vi "GUI_Bella_Control_Center.vi"() -> ()   [LabVIEW 2020]
uses:
  Shared/GUI_Template/GUI_master/tcp_new_data_event.ctl
  Shared/GUI_Template/GUI_master/tcp new data cluster.ctl
  GUI_TestStand/Fire button.ctl
  Device Drivers/DG645/subVIs/TriggerSource_TypDef.ctl
  <vilib>/Utility/config.llb/Write Key (I32).vi
  <vilib>/Platform/browser.llb/Open URL in Default Browser (string).vi
  <vilib>/Analysis/NI_AALBase.lvlib
  <vilib>/Utility/config.llb/NI_LVConfig.lvlib
panel:
  in  "JetOnTime":dbl=0.001 format="%#_6p"
  in  "Position.Channel 3::25":dbl caption="SMFiber (35.6in, 1out)" min=1.0 max=50.0 format="%.1f"
  in  "GasJetOn":bool
  in  "SendExptCmds":bool
  in  "ShotControl":bool
  in  "Thales.DIAG_CU_Output_Percent_1::37":dbl caption="Amp2 att (%)" min=1.0 max=100.0 step=500.0 format="%.2f"
  in  "GUIdevice 37":string="SVE-LT-Thales"
  in  "Pressure.device 1::39":dbl caption="Backing pressure" min=0.0 max=314.0 format="%.3f"
  in  "GUIdevice 39":string="PRC-PL1-HighPressure"
  in  "Scan":T1(ring)
  in  "LogTable":bool
  in  "New Google\nExpLog for new day?":bool=TRUE
  out "standard output":string
  in  "Create Log":bool caption="LogTable"
  in  "GUIdevice 38":string="STAGE-2BL-Compressor"
  in  "Position.Axis 1::38":dbl caption="Comp2 Translation" min=0.0 max=20.0 format="%.3f"
  in  "Position.Channel 5::31":T2(ring) caption="FROG foil"
  in  "Position.Channel 2::31":T2(ring) caption="Little Rick"
  in  "AnalogOutput.Channel 1::36":dbl caption="M4A att (V)" min=0.0 max=5.0 step=500.0 format="%.2f"
  in  "GUIdevice 36":string="ATT-2BL-M4A"
  in  "GUIdevice 35":string="ATT-2BL-DM"
  in  "AnalogOutput.Channel 1::35":dbl caption="2BL DM att (V)" min=0.0 max=5.0 step=500.0 format="%.2f"
  in  "Step size 2":dbl=20.0 caption="Step size" min=-22.0 max=22.0
  in  "Position.Axis 4::34":dbl caption="OFI Holy V F8" min=-100000.0 max=100000.0 step=500.0
  in  "Position.Axis 3::34":dbl caption="OFI Holy H F7" min=-100000.0 max=100000.0 step=500.0
  in  "Position.Axis 2::34":dbl caption="Axicon V F6" min=-100000.0 max=100000.0 step=500.0
  in  "Position.Axis 1::34":dbl caption="Axicon H F5" min=-100000.0 max=100000.0 step=500.0
  in  "GUIdevice 34":string="MCD-PL1-picosOFI2"
  in  "Position.Axis 4::33":dbl caption="BesselM1 V F4" min=-100000.0 max=100000.0 step=500.0
  in  "Position.Axis 3::33":dbl caption="BesselM1 H F3" min=-100000.0 max=100000.0 step=500.0
  in  "Position.Axis 2::33":dbl caption="OFI Probe V F2" min=-100000.0 max=100000.0 step=500.0
  in  "Position.Axis 1::33":dbl caption="OFI Probe H F1" min=-100000.0 max=100000.0 step=500.0
  in  "GUIdevice 33":string="MCD-PL1-picosOFI1"
  in  "delay.Channel_B::32":dbl caption="jet open time" min=-0.1 max=0.1 format="%.3p"
  in  "delay.Channel_A::32":dbl caption="jet open" min=-0.1 max=0.1 format="%.3p"
  in  "GUIdevice 32":string="DDG-AA-SRSgasjet"
  in  "position::6":dbl caption="LPmode stage long (605 safe)" min=0.0 max=605.0 format="%.1f"
  in  "GUIdevice 6":string="STAGE-PL1-LPmodeLong"
  in  "EnableMotor::6":bool caption="LPmode motor \nstatus"
  in  "CapStatus":enum16{"out", "in", "Unknown"}(ring) caption="Cap"
  in  "position::4":dbl=-1.631e-06 caption="Capstage" min=0.0 max=600.0 format="%.1f"
  in  "GUIdevice 4":string="STAGE-PL1-Capstage1"
  out "Boolean 2":bool
  in  "GUIdevice 31":string="1WIRE-BELLA-Flipper"
  in  "Position.Channel 4::31":T2(ring) caption="PL1 Fiber"
  in  "Amplitude.Ch GH::10":dbl=-1.631e-06 caption="Shot Shutter V" min=0.5 max=5.0 format="%.1f"
  in  "Rate (Hz)":dbl=0.3
  out "Crystal2":enum16{"In", "Out", "Unknown"}(ring)
  out "Hex1posdesc":enum16{"guiding", "fiber ref", "Unknown"}(ring) caption="Hex1"
  in  "DigitalOutput.Channel 0::30":enum16{"off", "on"}(ring) caption="GVD Plunger"
  in  "GUIdevice 30":string="DAQ-PL1-GVD"
  in  "GUIdevice 29":string="MCD-HEAT-ESP0"
  in  "Position.Axis 2::29":dbl caption="Y" min=-5.0 max=25.0 format="%.4f"
  in  "Position.Axis 1::29":dbl caption="X" min=-5.0 max=25.0 format="%.4f"
  in  "wangle::28":dbl caption="w" min=-1.0 max=1.0 step=0.01 format="%.5f"
  in  "vangle::28":dbl caption="v" min=-5.0 max=5.0 step=0.01 format="%.5f"
  in  "uangle::28":dbl caption="u" min=-1.0 max=1.0 step=0.01 format="%.5f"
  in  "ypos::28":dbl caption="y" min=-2.0 max=8.0 step=0.01 format="%.5f"
  in  "zpos::28":dbl caption="z" min=-5.0 max=5.0 step=0.01 format="%.5f"
  in  "xpos::28":dbl caption="x" min=-0.5 max=0.5 step=0.01 format="%.5f"
  in  "GUIdevice 28":string="HEX-PL1-2"
  in  "delay.Channel_A::27":dbl caption="Disch timing both caps" min=-0.1 max=0.1 format="%.3p"
  out "Boolean":bool
  in  "amplitude.Channel_A::27":dbl caption="Caps Trig (V)" min=-3.0 max=4.0 format="%.2f"
  in  "GUIdevice 27":string="DDG-AA-SRS3"
  in  "GUIdevice 26":string="PRC-PL1-PressureAPL"
  in  "pressure::26":dbl caption="Cap2 Pressure (Torr)" min=0.0 max=50.0 format="%.2f"
  in  "Position.Channel 5::25":dbl caption="Wedge (43.5,2)" min=0.0 max=50.0 format="%.1f"
  in  "Position.Channel 4::25":dbl caption="ND2 (4,45)" min=-35.0 max=-12.0 format="%.1f"
  in  "Position.Channel 1::25":dbl caption="LPmode kicker (79in, 1out)" min=0.5 max=83.0 format="%.1f"
  in  "Position.Channel 2::25":dbl caption="XH (38.1,2)" min=0.0 max=30.0 format="%.1f"
  in  "Position.Channel 1::25":dbl caption="ND3 (4,45)" min=0.5 max=83.0 format="%.1f"
  out "Data.Channel 2::14":dbl caption="Flow US (sccm)" min=0.0 max=1000.0 format="%.1f"
  out "pressure2::5":dbl caption="PDR US (Torr)" min=-100.0 max=500.0 format="%.2f"
  in  "Data.Channel 2::11":dbl caption="Pressure US (Torr)" min=0.0 max=1000.0 format="%.2f"
  in  "GUIdevice 25":string="STAGE-PL1-Smaract"
  in  "Heater Alignment Directions":bool
  in  "Position.device 4::16":dbl caption="2Y" min=-40000000.0 max=40000000.0
  in  "Position.device 3::16":dbl caption="2X" min=-40000000.0 max=40000000.0
  in  "Position.device 2::16":dbl caption="1Y" min=-40000000.0 max=40000000.0
  in  "Position.device 1::16":dbl caption="1X" min=-40000000.0 max=40000000.0
  in  "Position.Axis 3::15":dbl caption="XY" min=-3.0 max=16.0 format="%.4f"
  in  "Position.Axis 2::15":dbl caption="Y" min=-3.0 max=17.0 format="%.4f"
  in  "Position.Axis 1::15":dbl caption="X" min=-3.0 max=13.0 format="%.4f"
  in  "GUIdevice 24":string="STAGE-HEAT-TL1"
  in  "Encoder position::23":dbl caption="position HPD2" min=0.0 max=600.0 format="%.1f"
  in  "position::3":dbl caption="position HPD" min=0.0 max=600.0 format="%.1f"
  in  "GUIdevice 23":string="STAGE-HPD-Far"
  in  "GUIdevice 22":string="MANPAR-BELLA-FireCont"
  in  "Allow Fire Continues":bool
  out "Fire continues Indicator":bool caption="firing"
  in  "Fire Button":T3=TRUE
  in  "Trigger.Source::10":T4 caption="SRS Trigger Mode"
  in  "value2::21":dbl=-1.631e-06 caption="Offset" min=-9999999.0 max=9999999.0 format="%.3p"
  in  "value1::21":dbl=-0.000129636 caption="Offset" min=-9999999.0 max=9999999.0 format="%#.4p"
  out "Absolute Heater timing":dbl caption="delay" format="%#.4p"
  out "Absolute discharge timing":dbl caption="delay from pk" format="%#.3p"
  in  "delay.Channel_A::19":dbl caption="Timing box" min=-0.1 max=0.1 format="%#.4p"
  in  "Delay.Ch E::17":dbl caption="Timing box" min=-0.1 max=0.1 format="%.3p"
  in  "value0::22":bool caption="Fire continuosly"
  in  "GUIdevice 21":string="MANPAR-BELLA-Timing"
  out "PWshutter Scanstart":string
  out "Heater Scanstart":string
  in  "position::18":enum16{"out", "in", "Unknown"}(ring) caption="Cap stage"
  in  "bigshuttermode::18":enum16{"Auto", "Manual"}(ring) caption="Heater shutter mode"
  in  "smallshuttermode::18":enum16{"Auto", "Manual"}(ring) caption="PW tel4 shutter mode"
  in  "smallshutterposition::18":enum16{"out", "in", "Unknown"}(ring) caption="PW tel4 shutter"
  in  "bigshutterposition::18":enum16{"out", "in", "Unknown"}(ring) caption="Heater shutter"
  in  "voltage::20":dbl caption="Discharge HV (kV)" min=0.0 max=40.0 format="%.2f"
  in  "GUIdevice 20":string="HV-PL1-Glassman"
  in  "SlaveValue::11":dbl caption="Slave Value (%)" min=0.0 max=200.0 format="%.1f"
  in  "Update offsets":bool caption="Update"
  in  "Offset Heater timing":dbl=-0.000129636 caption="Offset" format="%#.3p"
  in  "Offset discharge timing":dbl=-1.631e-06 caption="Offset" format="%#.3p"
  in  "GUIdevice 19":string="DDG-HEAT-SRS1"
  in  "GUIdevice 18":string="STAGE-PL1-Cap1"
  in  "GUIdevice 16":string="PICO-HEAT-1"
  in  "GUIdevice 15":string="MCD-HEAT-ESP1"
  in  "GUIdevice 17":string="DDG-AA-SRS0"
  out "error IO 2":errorcluster
  out "fire::10":string
  out "tcp data event":T5
  in  "UDP error message":string
  in  "GUIdevice 14":string="GAUGE-PL1-FlowStage1"
  in  "GUIdevice 13":string="DDG-AA-SRS2"
  in  "GUIdevice 7":string="MANPAR-PL1-BottlePressure"
  in  "parameter::2":string="parameter" caption="Manual parameter"
  in  "GUIdevice 2":string="MANPAR-BELLA-General"
  in  "GUIdevice 10":string="DDG-AA-ShotCntrl"
  in  "GUIdevice 5":string="GAUGE-PL1-Pressure"
  in  "GUIdevice 1":string="HEX-PL1-1"
  in  "GUIdevice 3":string="STAGE-HPD-Tel"
  in  "GUIdevice 11":string="PRC-PL1-Stage1"
  in  "Delay.Ch E::13":dbl caption="Discharge timing (s)" min=-0.1 max=0.2 format="%#_9p"
  out "Trans sigma":dbl format="%0.2f"
  out "Trans Mean":dbl format="%0.2f"
  out "Waveform Chart":dbl(graph)
  out "EnergyIn::2":dbl caption="Ein" min=0.0 max=0.0 format="%.1p"
  out "EnergyOut::12":dbl caption="Eout" min=0.0 max=0.0 format="%.1p"
  in  "EnergyTransmission::12":dbl caption="Etrans (%)" min=0.0 max=0.0
  in  "GUIdevice 12":string="EM-AA-Trans1"
  in  "<command>::1":bool caption="ABORT\nHEXAPOD"
  in  "Step size":dbl min=-22.0 max=22.0 format="%.5f"
  in  "wangle::1":dbl caption="w (F11 F12)" min=-6.0 max=6.0 step=0.01 format="%.5f"
  in  "vangle::1":dbl caption="v (F9 F10)" min=-6.0 max=6.0 step=0.01 format="%.5f"
  in  "uangle::1":dbl caption="u (F7 F8)" min=-6.0 max=6.0 step=0.01 format="%.5f"
  in  "ypos::1":dbl caption="y (F3 F4)" min=-20.0 max=10.0 step=0.01 format="%.5f"
  in  "zpos::1":dbl caption="z (PgU PgD)" min=-12.0 max=1.0 step=0.01 format="%.5f"
  in  "xpos::1":dbl caption="x (F1 F2)" min=-22.0 max=22.0 step=0.01 format="%.5f"
  in  "value::7":dbl caption="Bottle Pressure" min=0.0 max=1000.0
  in  "Pressure.device 1::6":dbl caption="Alicat Pressure" min=0.0 max=314.0 format="%.2f"
  in  "Position.Axis 1::9":dbl caption="Comp1 Translation" min=-50.0 max=50.0 format="%.3f"
  in  "GUIdevice 9":string="STAGE-1BL-Compression"
  out "Data.Channel 1::14":dbl caption="Flow DS (sccm)" min=0.0 max=1000.0 format="%.1f"
  in  "Data.Channel 1::11":dbl caption="Pressure DS (Torr)" min=0.0 max=1000.0 format="%.2f"
  out "pressure::5":dbl caption="PDR DS (Torr)" min=-100.0 max=500.0 format="%.2f"
  in  "Delay.Ch C::10":dbl caption="Jet timing (s)" min=-0.1 max=2.1 format="%#_6p"
  in  "stop":bool
  # "BELLA CONTROL CENTER"
  # "CAP"
  # "Hex2"
  # "HEXAPOD"
  # "PICOS"
  # "DG"
  # "HEXAPOD 2"
  # "Energy"
  # "GAS JET"
  # "Scan"
  # "Discharge timing (s)"
  # "Send only. Does not read"
  # "1wire"
  # "Jet"
  # "Heater timing (s)"
  # "\"-x\" is laser propagation direction"
  # "HPD Stage"
  # "PL1 stages"
  # "Heater Alignment"
  # "Atttenuate"
  # "Heat ESP0"
  # "Heat ESP1"
  # "Compressors"
  # "Heat Pico"
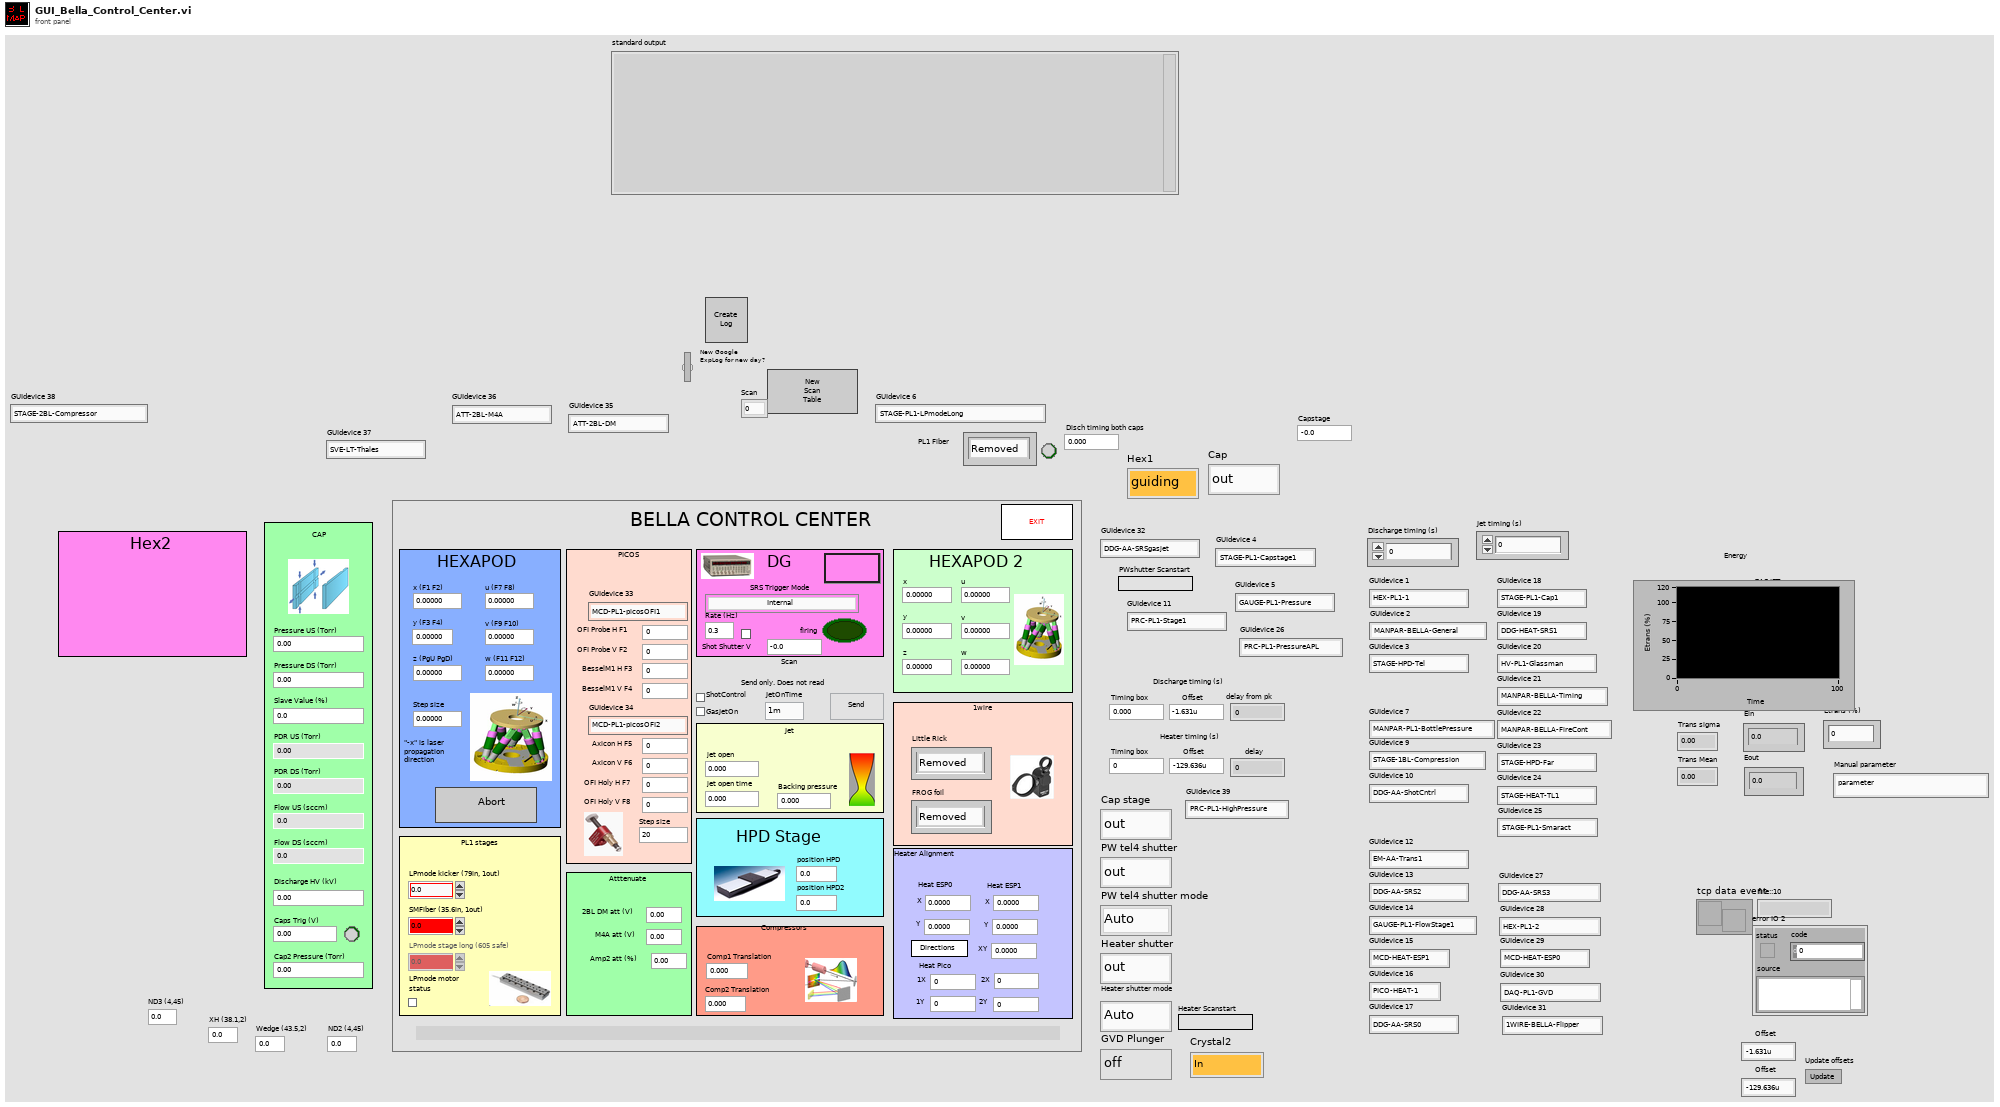
[diagram p1: front panel]
types:
  T1 = enum16{"0", "1", "2", "3", "4", "5", "6", "7", "8", "9", "10", "11", "12", "13", "14", "15", "16", "17", "18", "19", "20", "21", "22", "23", "24", "25", "26", "27", "28", "29", "30", "31", "32", "33", "34", "35", "36", "37", "38", "39", "40", "41", "42", "43", "44", "45", "46", "47", "48", "49", "50", "51", "52", "53", "54", "55", "56", "57", "58", "59", "60", "61", "62", "63", "64", "65", "66", "67", "68", "69", "70", "71", "72", "73", "74", "75", "76", "77", "78", "79", "81", "82", "83", "84", "85", "86", "87", "88", "89", "90", "91", "92", "93", "94", "95", "96", "97", "98", "99", ""}
  T2 = enum16{"Removed", "Inserted", "Unknown", "Moving"}
  T3 = typedef "Fire button.ctl" = bool
  T4 = typedef "TriggerSource_TypDef.ctl" = enum16{"Internal", "External rising edges", "External falling edges", "Single shot external rising edges", "Single shot external falling edges", "Single shot", "Line"}
  T5 = typedef "tcp_new_data_event.ctl" = refnum<user-event>
  T6 = typedef "tcp new data cluster.ctl" = cluster{"EventEnum":enum16{"new data", "connection status update"}, "Device name":string}
  T7 = enum8{"Enabled", "Disabled", "Disabled and Grayed Out"}
  T8 = enum32{"invalid app kind", "Development System", "Run Time System", "Student Edition", "Embedded LabVIEW", "Evaluation", "Custom"}
  T9 = enum32{"Invalid", "Standard", "Closed", "Hidden", "Minimized", "Maximized"}
  T10 = typedef "imagedata.ctl" = cluster{"image type":i32, "image depth":i32, "image":u8[], "mask":u8[], "colors":u32[], "Rectangle":cluster{"left":i16, "top":i16, "right":i16, "bottom":i16}}
  T11 = typedef "NI_LVConfig.lvlib/Config Data RefNum.ctl" = refnum<k1>
  T12 = cluster{"Core":cluster{"Current VI Reference":refnum<vi>, "Close Panel on Exit?":bool}, "Heater timing offset":dbl, "Discharge timing offset":dbl, "Jet trigger":bool, "Tik1":u32, "Tik2":u32, "Fire Continues Allowed":bool}
  T13 = cluster{"Current VI Reference":refnum<vi>, "Close Panel on Exit?":bool}
  T14 = typedef "mysql_authentication.ctl" = cluster{"User":string, "Password":string, "Database":string}
  T15 = cluster{"Port":u16, "IP Address":string, "Authentication":T14}
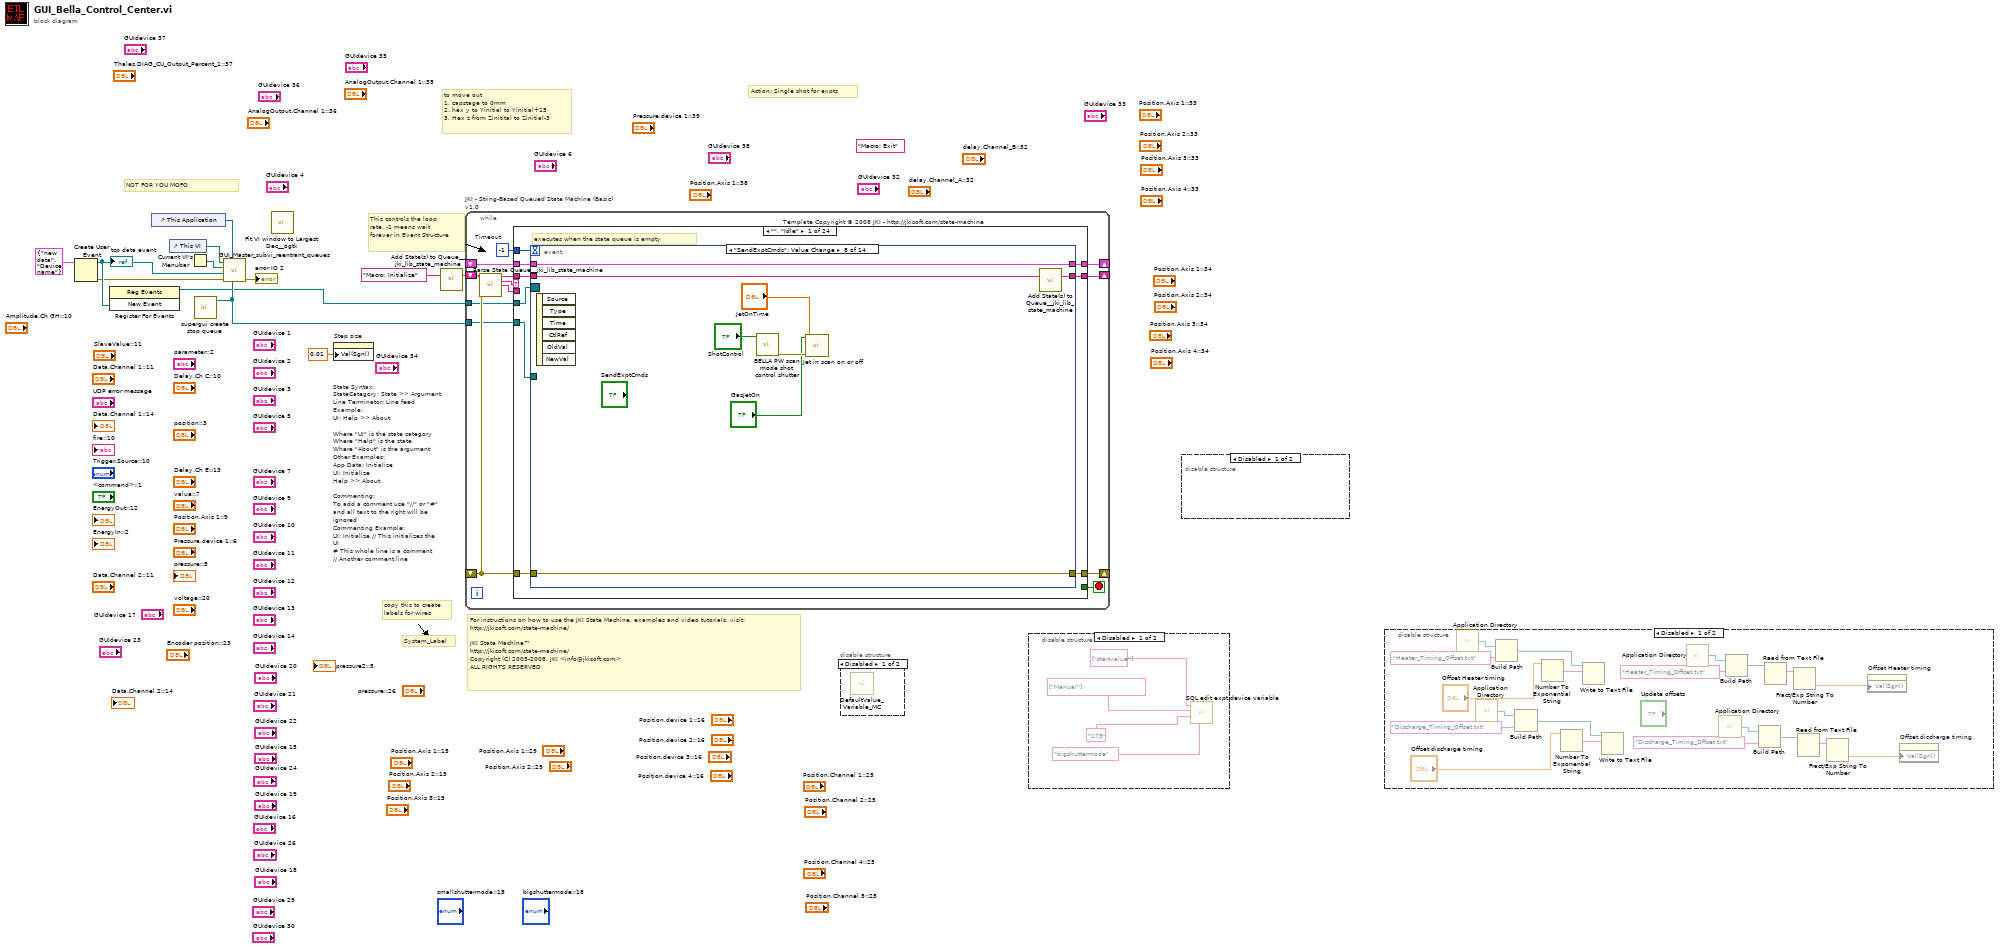
[diagram p0: block diagram]
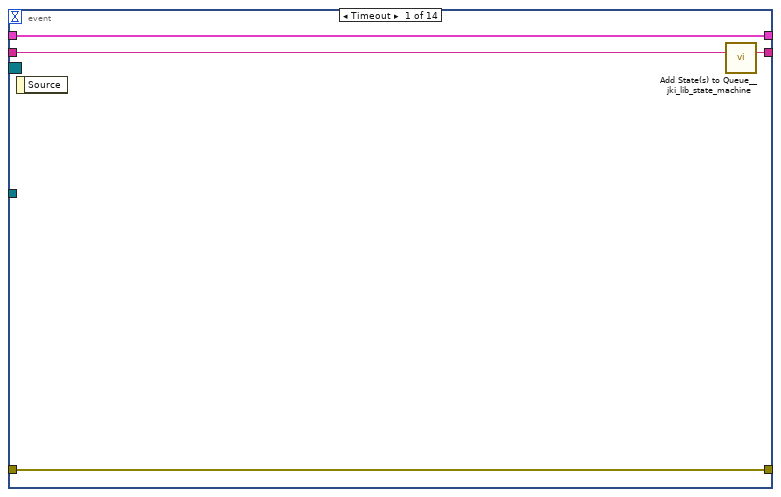
[diagram p6: hidden frame]
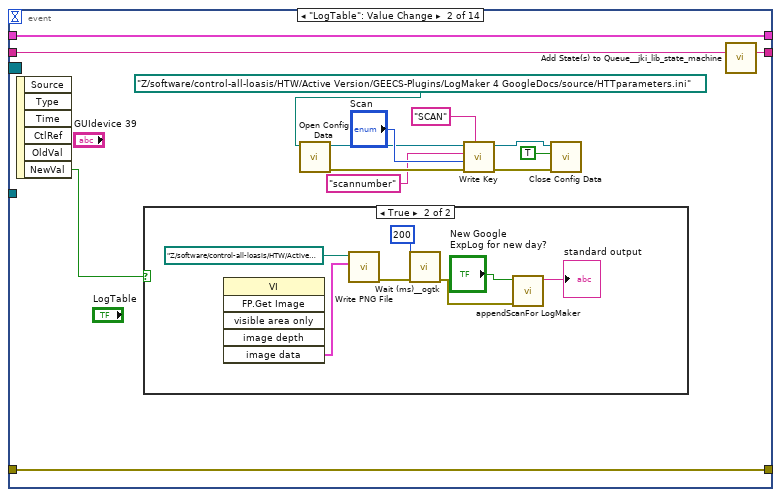
[diagram p7: hidden frame]
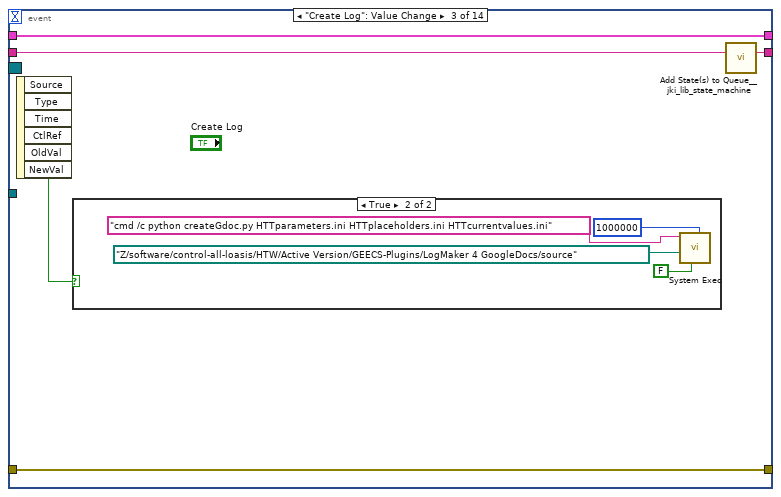
[diagram p9: hidden frame]
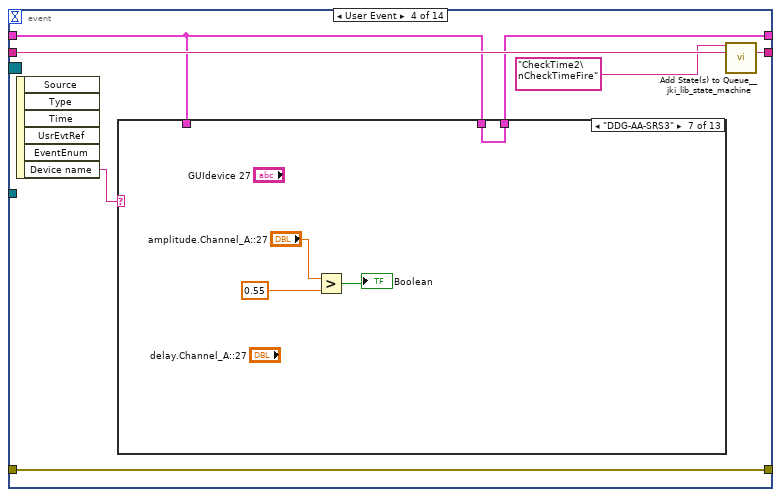
[diagram p11: hidden frame]
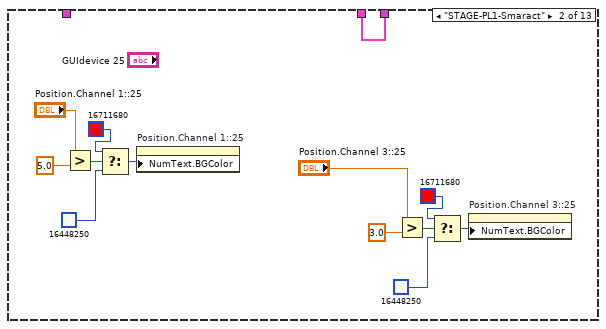
[diagram p13: hidden frame]
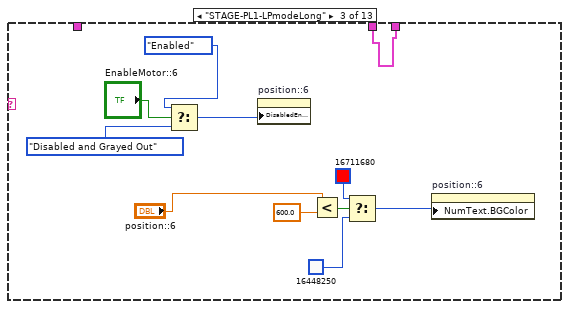
[diagram p14: hidden frame]
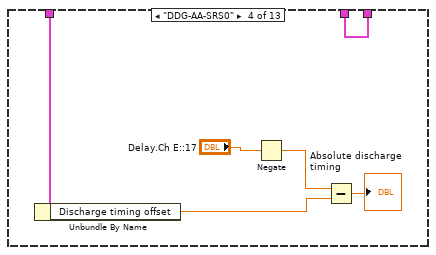
[diagram p15: hidden frame]
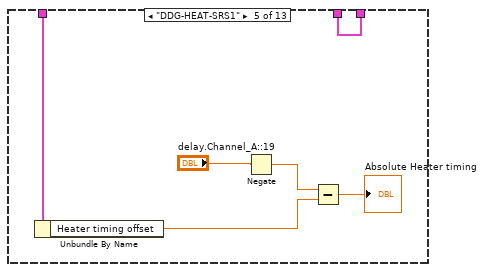
[diagram p16: hidden frame]
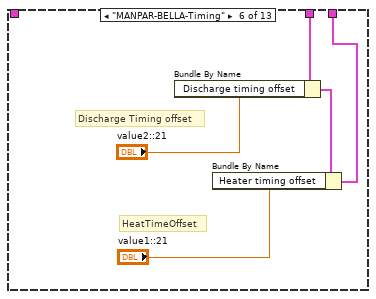
[diagram p17: hidden frame]
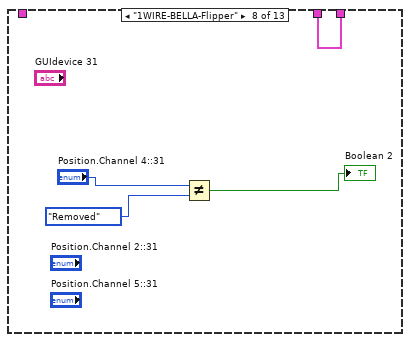
[diagram p18: hidden frame]
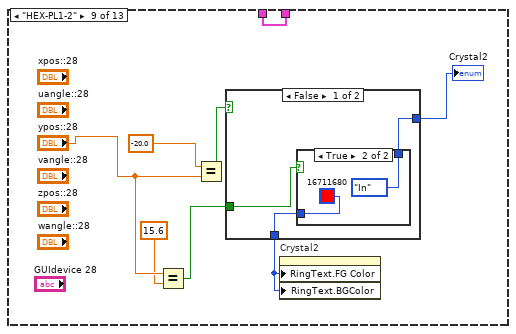
[diagram p19: hidden frame]
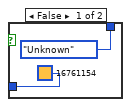
[diagram p20: hidden frame]
diagram:
  (unwired) "Macro: Exit"
  # "Action: Single shot for expts"
  # "to move out\n1. capstage to 0mm\n2. hex y to Yinitial to Yinitial+15\n3. Hex z from Zinitital to Zinitial-3"
  # "For instructions on how to use the JKI State Machine, examples and video tutorials, visit:\nhttp://jkisoft.com/state-machine/\n\nJKI State Machine™\nhttp://jkisoft.com/state-machine/\nCopyright (C) 2005-2008, JKI <info@jkisoft.com>\nALL RIGHTS RESERVED"
  # "State Syntax:\nStateCategory: State >> Argument\nLine Terminator: Line feed\nExample:\nUI: Help >> About\n\nWhere \"UI\" is the state category\nWhere \"Help\" is the state\nWhere \"About\" is the argument\nOther Examples:\nApp Data: Initialize\nUI: Initialize\nHelp >> About\n\nCommenting:\nTo add a comment use \"//\" or \"#\" and all text to the right will be ignored\nCommenting Example:\nUI: Initialize // This initializes the UI\n# This whole line is a comment\n// Another comment line"
  # "copy this to create labels for wires"
  # "This controls the loop rate. -1 means wait forever in Event Structure"
  # "System_Label"
  # "NOT FOR YOU MOFO"
  n1 = Create User Event(user event datatype=T6 {"EventEnum"=enum."new data", "Device name"="Device name"} ("New Event")) -> (user event=w11:refnum<user-event>, error out=w10:errorcluster)  [unwired: 1 in]
  "tcp data event" <- w11
  n2 = register-events(w11) -> (reference out=w1:refnum<event-registration>)  [unwired: 2 in, 1 out]
  n3 = control-ref of="This Application"() -> (w12:refnum<vi>)
  n4 = control-ref of="This VI"() -> (w5:refnum<vi>)
  n5 = Current VI's Menubar() -> (w8:refnum<k9>)
  n6 = call "supergui create stop queue.vi"() -> ("STOP Queue out"=w2:refnum<queue>)  [unwired: 11 in]
  n7 = call "GUI_Master_subvi_reentrant_queues.vi"("STOP Queue in"=w2, "This Application"=w12, "error in (no error)"=w10, "tcp data event"=w11, "Caller menu reference"=w8, "Caller VI ref"=w5) -> ("error out"=→"error IO 2":errorcluster)  [unwired: 5 in]
  n8 = call <userlib>:"Fit VI window to Largest Dec__ogtk.vi"() -> ()  [unwired: 6 in, 2 out]
  n9 = property on="Step size" class="DigNum (strict)"("Val(Sgnl)"=0.01 ("Value (Signaling)")) -> ()  [unwired: 2 in, 2 out]
  n10 = call <vilib>:"Add State(s) to Queue__jki_lib_state_machine.vi"("State(s) in (\"\")"="Macro: Initialize") -> ("States Out"=w3:string)  [unwired: 14 in]
  n11 = while "JKI - String-Based Queued State Machine (Basic) v1.0" {
    shift-right: [w18] -> _
    shift-left: _ -> [w17]
    shift-right: [w21] -> _
    shift-left: _ -> [w15]
    shift-right: [w20] -> _
    shift-left: w3 -> [w22]
    tunnel: w1 -> [w14]
    tunnel: w2 -> [w13]
    stop <- w19 stop-if-true
    w16 = -1  # Timeout
    # "Template Copyright © 2008 JKI - http://jkisoft.com/state-machine"
    n12 = call <vilib>:"Parse State Queue__jki_lib_state_machine.vi"("State Queue"=w22, "Error In (no error)"=w15) -> ("Remaining States"=w24:string, "Current State"=w25:string, "Arguments"=w23:string)  [unwired: 11 in]
    n13 = case shown="\"\", \"Idle\"" w25 {
      selector: w25 -> [_ _ w291 _ _ _ _ _ _ _ _ _ _ _ _ _ _ _ _ _ _ _ _ _]
      tunnel: w24 -> [w34 w290 w295 w313 w319 w324 w328 w339 w345 w349 w353 w359 w370 w396 w401 w414 w418 w437 w448 w460 w472 w481 w499 w520]
      tunnel: w23 -> [_ _ _ _ _ _ _ _ _ _ _ w354 w364 _ _ _ _ _ _ _ _ _ w492 _]
      tunnel: w17 -> [w32 w287 w293 w304 w316 w322 w325 _ w340 w346 w351 w357 w366 w393 w398 w411 w415 w425 w444 w454 w469 w479 w497 w517]
      tunnel: [w31 w288 w297 w310 errorcluster {"status"=FALSE, "code"=0, "source"=""} ("error out") w321 w326 w336 w341 w347 w350 w355 w367 w394 w399 w412 w416 w435 w442 w449 w470 w476 w493 w518] -> w21
      tunnel: w15 -> [w30 w288 w296 w310 w315 w321 w326 w336 w342 w347 w350 w356 w368 w394 w399 w412 w416 w435 w446 w450 w470 w477 w494 w518]
      tunnel: [w33 w289 w294 w312 w318 w323 w327 w338 w344 w348 w352 w358 w369 w395 w400 w413 w417 w436 w447 w459 w471 w480 w498 w519] -> w20
      tunnel: [_ _ _ _ _ TRUE _ _ _ _ _ _ _ _ _ _ _ _ _ _ _ _ _ _] -> w19
      tunnel: [w26 w287 w293 w311 w316 w322 w325 w337 w340 w346 w351 w357 w366 w393 w398 w411 w415 w434 w444 w453 w468 w479 w497 w517] -> w18
      tunnel: w16 -> [w29 _ _ _ _ _ _ _ _ _ _ _ _ _ _ _ _ _ _ _ _ _ _ _]
      tunnel: w14 -> [w28 _ _ _ _ _ _ _ _ _ _ _ _ _ _ _ _ _ _ _ _ _ _ _]
      tunnel: w13 -> [w27 _ _ _ _ _ _ _ _ _ _ _ _ _ _ w403 _ _ _ _ _ _ _ _]
      frame "", "Idle" {
        # "executes when the state queue is empty"
        n14 = event shown="[7] \"SendExptCmds\": Value Change" {
          selector: w28 -> [_ _ _ _ _ _ _ _ _ _ _ _ _ _]
          dyn-events: _ -> [_ _ _ _ _ _ _ _ _ _ _ _ _ _]
          timeout: w29 -> [_ _ _ _ _ _ _ _ _ _ _ _ _ _]
          tunnel: w34 -> [w38 w52 w64 w75 w196 w201 w211 w219 w227 w236 w259 w273 w280 w286]
          tunnel: [w37 w51 w63 w74 w195 w202 w212 w220 w227 w235 w259 w273 w280 w285] -> w33
          tunnel: w32 -> [w35 w49 w61 w70 w193 w200 w214 w222 w226 w238 w260 w274 w279 w283]
          tunnel: [w36 w50 w62 w73 w194 w203 w213 w221 w224 w241 w258 w272 w278 w284] -> w31
          tunnel: w30 -> [w36 w50 w62 w73 w194 w203 w213 w221 w225 w240 w258 w272 w278 w284]
          tunnel: [w35 w49 w61 w69 w193 w200 w214 w222 w226 w239 w260 w274 w279 w283] -> w26
          tunnel: w27 -> [_ _ _ _ _ _ _ _ _ _ _ _ _ _]
          event Timeout {
            n15 = event-data() -> ()  [unwired: 1 in, 1 out]
            n16 = call <vilib>:"Add State(s) to Queue__jki_lib_state_machine.vi"("State(s) in (\"\")"=w38) -> ("States Out"=w37:string)  [unwired: 14 in]
          }
          event "LogTable": Value Change {
            n17 = event-data() -> ("NewVal"=w39:bool)  [unwired: 1 in, 5 out]
            n18 = case shown="True" w39 {
              frame False {
              }
              frame True {
                n19 = invoke class="VI" method="FP.Get Image"() -> ("image data"=w59:T10)  [unwired: 6 in, 5 out]
                n20 = call <vilib>:"Write PNG File.vi"("image data"=w59, "path to PNG file"=path "Z:/software/control-all-loasis/HTW/Active Version/GEECS-Plugins/LogMaker 4 GoogleDocs/source/frontpanel.png" ("report file path")) -> ("error out"=w54:errorcluster)  [unwired: 8 in, 1 out]
                n21 = call <userlib>:"Wait (ms)__ogtk.vi"("error in (no error)"=w54, "milliseconds to wait"=u32 200 ("millisecond timer value")) -> ("error out"=w53:errorcluster)  [unwired: 8 in, 1 out]
                n22 = call "appendScanFor LogMaker.vi"("error in (no error)"=w53, "New Google\nExpLog for new day?"="New Google\nExpLog for new day?") -> ("standard output"=→"standard output":string)  [unwired: 9 in]
              }
            }
            n23 = call <vilib>:"Open Config Data.vi"("configuration file path"=path "Z:/software/control-all-loasis/HTW/Active Version/GEECS-Plugins/LogMaker 4 GoogleDocs/source/HTTparameters.ini") -> ("error out"=w46:errorcluster, "refnum"=w44:T11)  [unwired: 8 in, 1 out]
            n24 = call-poly <vilib>:"Write Key.vi"("section"="SCAN", "error in (no error)"=w46, "value"="Scan", "key"="scannumber", "refnum"=w44) -> ("error out"=w47:errorcluster, "refnum out"=w45:T11)  [unwired: 4 in, 1 out]
            n25 = call <vilib>:"Close Config Data.vi"("error in (no error)"=w47, "write file if changed (T)"=TRUE, "refnum"=w45) -> ()  [unwired: 7 in, 2 out]
            n26 = call <vilib>:"Add State(s) to Queue__jki_lib_state_machine.vi"("State(s) in (\"\")"=w52) -> ("States Out"=w51:string)  [unwired: 14 in]
          }
          event "Create Log": Value Change {
            n27 = event-data() -> ("NewVal"=w60:bool)  [unwired: 1 in, 5 out]
            n28 = case shown="True" w60 {
              frame False {
              }
              frame True {
                n29 = call <vilib>:"System Exec.vi"("expected output size  (4096)"=u32 1000000, "run minimized? (F)"=FALSE, "working directory"=path "Z:/software/control-all-loasis/HTW/Active Version/GEECS-Plugins/LogMaker 4 GoogleDocs/source", "command line"="cmd /c python createGdoc.py HTTparameters.ini HTTplaceholders.ini HTTcurrentvalues.ini") -> ()  [unwired: 4 in, 4 out]
              }
            }
            n30 = call <vilib>:"Add State(s) to Queue__jki_lib_state_machine.vi"("State(s) in (\"\")"=w64) -> ("States Out"=w63:string)  [unwired: 14 in]
          }
          event User Event {
            n31 = event-data() -> ("Device name"=w72:string)  [unwired: 1 in, 5 out]
            n32 = case shown="\"DDG-AA-SRS3\"" w72 {
              tunnel: w70 -> [_ _ _ w103 w109 _ _ _ _ _ _ _ _]
              tunnel: w70 -> [w76 w89 w100 w101 w107 w116 w120 w122 w133 w147 w166 w171 w189]
              tunnel: [w76 w89 w100 w101 w107 w113 w120 w122 w133 w147 w166 w171 w189] -> w69
              frame "False", Default {
              }
              frame "STAGE-PL1-Smaract" {
                n33 = Greater?(x="Position.Channel 1::25", y=5.0) -> (0:w86:bool)
                n34 = Select(t=u32 16711680, s=w86, f=u32 16448250) -> (s? t:f=w83:u32)
                n35 = property on="Position.Channel 1::25" class="DigNum (strict)"("NumText.BGColor"=w83) -> ()  [unwired: 2 in, 2 out]
                n36 = Greater?(x="Position.Channel 3::25", y=3.0) -> (0:w79:bool)
                n37 = Select(t=u32 16711680, s=w79, f=u32 16448250) -> (s? t:f=w82:u32)
                n38 = property on="Position.Channel 3::25" class="DigNum (strict)"("NumText.BGColor"=w82) -> ()  [unwired: 2 in, 2 out]
              }
              frame "STAGE-PL1-LPmodeLong" {
                n39 = Select(t=T7."Enabled" ("Disabled"), s="EnableMotor::6", f=T7."Disabled and Grayed Out" ("Disabled")) -> (s? t:f=w90:T7)
                n40 = property on="position::6" class="DigNum (strict)"("DisabledEnum"=w90) -> ()  [unwired: 2 in, 2 out]
                n41 = Less?(x="position::6", y=600.0) -> (x < y?=w99:bool)
                n42 = Select(t=u32 16711680, s=w99, f=u32 16448250) -> (s? t:f=w94:u32)
                n43 = property on="position::6" class="DigNum (strict)"("NumText.BGColor"=w94) -> ()  [unwired: 2 in, 2 out]
              }
              frame "DDG-AA-SRS0" {
                n44 = Unbundle By Name(w103) -> ("Discharge timing offset"=w102:dbl)
                n45 = Negate(x="Delay.Ch E::17") -> (-x=w104:dbl)
                n46 = Subtract(x=w104, y=w102) -> (x-y=→"Absolute discharge timing":dbl)
              }
              frame "DDG-HEAT-SRS1" {
                n47 = Unbundle By Name(w109) -> ("Heater timing offset"=w108:dbl)
                n48 = Negate(x="delay.Channel_A::19") -> (-x=w110:dbl)
                n49 = Subtract(x=w110, y=w108) -> (x-y=→"Absolute Heater timing":dbl)
              }
              frame "MANPAR-BELLA-Timing" {
                # "HeatTimeOffset"
                # "Discharge Timing offset"
                n50 = Bundle By Name(cluster=w116, "Discharge timing offset"="value2::21") -> (w114:T12)
                n51 = Bundle By Name(cluster=w114, "Heater timing offset"="value1::21") -> (w113:T12)
              }
              frame "DDG-AA-SRS3" {
                n52 = Greater?(x="amplitude.Channel_A::27", y=0.55) -> (0:→"Boolean":bool)
              }
              frame "1WIRE-BELLA-Flipper" {
                n53 = Not Equal?(x="Position.Channel 4::31", y=T2."Removed" ("Position.Channel 4::31")) -> (x != y?=→"Boolean 2":bool)
              }
              frame "HEX-PL1-2" {
                n54 = Equal?(x="ypos::28", y=15.6) -> (x = y?=w127:bool)
                n55 = Equal?(x=-20.0 ("y"), y="ypos::28") -> (x = y?=w131:bool)
                n56 = case shown="False" w131 {
                  tunnel: [w136 enum16{"In", "Out"}."Out" ("sdfsdfs 2")] -> w126
                  tunnel: [w134 u32 16185078] -> w130
                  tunnel: w127 -> [w135 _]
                  frame False {
                    n57 = case shown="True" w135 {
                      tunnel: [enum16{"In", "Out", "Unknown"}."Unknown" ("sdfsdfs 2") enum16{"In", "Out"}."In" ("sdfsdfs 2")] -> w136
                      tunnel: [u32 16761154 ("Color Box") u32 16711680] -> w134
                      frame False {
                      }
                      frame True {
                      }
                    }
                  }
                  frame True {
                  }
                }
                "Crystal2" <- w126
                n58 = property on="Crystal2" class="Enum (strict)"("RingText.FG Color"=w130, "RingText.BGColor"=w130) -> ()  [unwired: 2 in, 2 out]
              }
              frame "HEX-PL1-1" {
                n59 = call "Hexapod1check.vi"("zpos::1"="zpos::1", "ypos::1"="ypos::1") -> ("sdfsdfs"=w145:enum16{"guiding", "fiber ref", "Unknown"})  [unwired: 9 in]
                "Hex1posdesc" <- w145
                n60 = case shown="\"Unknown\"" w145 {
                  tunnel: [u32 16448250 u32 16711680 u32 16761154] -> w146
                  frame "guiding", Default {
                  }
                  frame "fiber ref" {
                  }
                  frame "Unknown" {
                  }
                }
                n61 = property on="Hex1posdesc" class="Enum (strict)"("RingText.FG Color"=w146, "RingText.BGColor"=w146) -> ()  [unwired: 2 in, 2 out]
                n62 = case shown="\"Unknown\"" w145 {
                  tunnel: [w154 w158 enum16{"out", "in", "Unknown"}."Unknown" ("CapStatus")] -> w143
                  tunnel: "position::4" -> [w153 w161 _]
                  frame "guiding", Default {
                    n63 = In Range and Coerce(upper limit=25.05, x=w153, lower limit=24.95) -> (In Range?=w150:bool)  [unwired: 1 out]
                    n64 = Select(t=enum16{"out", "in", "Unknown"}."in" ("CapStatus"), s=w150, f=enum16{"out", "in", "Unknown"}."Unknown" ("CapStatus")) -> (s? t:f=w154:enum16{"out", "in", "Unknown"})
                  }
                  frame "fiber ref" {
                    n65 = Equal To 0?(x=w161) -> (x = 0?=w160:bool)
                    n66 = Select(t=enum16{"out", "in", "Unknown"}."out" ("CapStatus"), s=w160, f=enum16{"out", "in", "Unknown"}."Unknown" ("CapStatus")) -> (s? t:f=w158:enum16{"out", "in", "Unknown"})
                  }
                  frame "Unknown" {
                  }
                }
                n67 = local write "CapStatus"(w143) -> ()
              }
              frame "EM-AA-Trans1" {
                n68 = property on="Waveform Chart" class="WFChart (strict)"() -> ("History Data"=w169:dbl[])  [unwired: 2 in, 2 out]
                n69 = call <vilib>:"Std Deviation and Variance.vi"("X"=w169) -> ("mean"=→"Trans Mean":dbl, "standard deviation"=→"Trans sigma":dbl)  [unwired: 1 in, 1 out]
                "Waveform Chart" <- "EnergyTransmission::12"
              }
              frame "STAGE-PL1-Cap1" {
                n70 = case shown="\"in\"" "position::18" {
                  tunnel: [u32 16448250 u32 16711680 u32 13816530] -> w173
                  frame "out", Default {
                  }
                  frame "in" {
                  }
                  frame "Unknown" {
                  }
                }
                n71 = case shown="\"out\", Default" "smallshutterposition::18" {
                  tunnel: [u32 16711680 u32 16448250 u32 13816530] -> w175
                  frame "out", Default {
                  }
                  frame "in" {
                  }
                  frame "Unknown" {
                  }
                }
                n72 = case shown="\"Unknown\"" "bigshutterposition::18" {
                  tunnel: [u32 16711680 u32 16448250 u32 13816530] -> w177
                  frame "out", Default {
                  }
                  frame "in" {
                  }
                  frame "Unknown" {
                  }
                }
                n73 = property on="position::18" class="Enum (strict)"("RingText.FG Color"=w173, "RingText.BGColor"=w173) -> ()  [unwired: 2 in, 2 out]
                n74 = property on="smallshutterposition::18" class="Enum (strict)"("RingText.FG Color"=w175, "RingText.BGColor"=w175) -> ()  [unwired: 2 in, 2 out]
                n75 = property on="bigshutterposition::18" class="Enum (strict)"("RingText.FG Color"=w177, "RingText.BGColor"=w177) -> ()  [unwired: 2 in, 2 out]
              }
              frame "DAQ-PL1-GVD" {
                n76 = case shown="\"off\", Default" "DigitalOutput.Channel 0::30" {
                  tunnel: [u32 16777225 u32 16711680] -> w188
                  frame "off", Default {
                  }
                  frame "on" {
                  }
                }
                n77 = property on="DigitalOutput.Channel 0::30" class="Enum (strict)"("RingText.FG Color"=w188, "RingText.BGColor"=w188) -> ()  [unwired: 2 in, 2 out]
              }
            }
            n78 = call <vilib>:"Add State(s) to Queue__jki_lib_state_machine.vi"("State(s) in Front (\"\")"="CheckTime2\nCheckTimeFire" ("State(s) in Front (\"\")"), "State(s) in (\"\")"=w75) -> ("States Out"=w74:string)  [unwired: 13 in]
          }
          event "stop": Value Change {
            # "Exit Button Value Change (pressed) Event\n(this executes Macro: Exit to terminate the VI)"
            n79 = event-data() -> ()  [unwired: 1 in, 6 out]
            n80 = call <vilib>:"Add State(s) to Queue__jki_lib_state_machine.vi"("State(s) in Front (\"\")"="Macro: Exit", "State(s) in (\"\")"=w196) -> ("States Out"=w195:string)  [unwired: 13 in]
          }
          event "CapStatus": Value Change {
            n81 = event-data() -> ("OldVal"=w197:enum16{"out", "in", "Unknown"}, "NewVal"=w199:enum16{"out", "in", "Unknown"})  [unwired: 1 in, 4 out]
            n82 = case shown="\"in\", Default" w197 {
              tunnel: w199 -> [_ w207]
              tunnel: [_ w204] -> w198
              frame "Unknown" {
              }
              frame "in", Default {
                n83 = case shown="\"in\"" w207 {
                  tunnel: ["Out" ("Arguments (\"\")") "In" ("Arguments (\"\")")] -> w205
                  frame "out", Default {
                  }
                  frame "in" {
                  }
                }
                n84 = call <vilib>:"Build State String with Arguments__JKI_lib_State_Machine.vi"("Arguments (\"\")"=w205, "State"="Action: MoveCap" ("State(s) in Front (\"\")")) -> ("State with Arguments"=w204:string)  [unwired: 4 in]
              }
            }
            n85 = call <vilib>:"Add State(s) to Queue__jki_lib_state_machine.vi"("State(s) in Front (\"\")"=w198, "State(s) in (\"\")"=w201) -> ("States Out"=w202:string)  [unwired: 13 in]
          }
          event Value Change {
            n86 = event-data() -> ()  [unwired: 1 in, 6 out]
            n87 = call <vilib>:"Add State(s) to Queue__jki_lib_state_machine.vi"("State(s) in Front (\"\")"="Action: Fire" ("State(s) in Front (\"\")"), "State(s) in (\"\")"=w211) -> ("States Out"=w212:string)  [unwired: 13 in]
          }
          event "SendExptCmds": Value Change {
            n88 = event-data() -> ()  [unwired: 1 in, 6 out]
            n89 = call "BELLA PW scan mode shot control shutter.vi"("ScanShotControl"="ShotControl") -> ("error out"=w217:errorcluster)  [unwired: 10 in]
            n90 = call "Jet in scan on or off.vi"("error in (no error)"=w217, "gas jet on time"="JetOnTime", "GasJetOn"="GasJetOn") -> ()  [unwired: 8 in, 1 out]
            n91 = call <vilib>:"Add State(s) to Queue__jki_lib_state_machine.vi"("State(s) in (\"\")"=w219) -> ("States Out"=w220:string)  [unwired: 14 in]
          }
          event "Heater Alignment Directions": Value Change {
            n92 = event-data() -> ()  [unwired: 1 in, 6 out]
            n93 = case shown="True" "Heater Alignment Directions" {
              tunnel: w225 -> [w228 w231]
              tunnel: [w228 w230] -> w224
              frame False {
              }
              frame True {
                n94 = call-poly <vilib>:"Open URL in Default Browser.vi"("error in (no error)"=w231, "URL"="https://docs.google.com/document/d/1RMZp6W8Kkog2nkTymSjyZ2bh9D7Vo4bxhvGgn3Ut4KE/edit") -> ("error out"=w230:errorcluster)  [unwired: 4 in, 1 out]
              }
            }
          }
          event "Allow Fire Continues": Value Change {
            n95 = event-data() -> ()  [unwired: 1 in, 6 out]
            n96 = Unbundle By Name(w238) -> ("Fire Continues Allowed"=w237:bool)
            n97 = case shown="True" "Allow Fire Continues" {
              tunnel: [w242 w249] -> w241
              tunnel: "Allow Fire Continues" -> [_ w248]
              tunnel: w240 -> [w242 w247]
              tunnel: w237 -> [w243 w246]
              tunnel: [w243 w244] -> w233
              tunnel: [_ "Initilize Fire Continues" ("State(s) in Front (\"\")")] -> w232
              frame False {
              }
              frame True {
                n98 = case shown="False" w246 {
                  tunnel: [w255 w256] -> w249
                  tunnel: w248 -> [w254 _]
                  tunnel: w247 -> [w253 w256]
                  tunnel: [w250 FALSE] -> w244
                  frame False {
                    n99 = call "Password"("Enable"=w254, "error in (no error)"=w253) -> ("Password"=w252:string, "error out"=w255:errorcluster)  [unwired: 15 in, 1 out]
                    n100 = Equal?(x=w252, y="fire") -> (x = y?=w250:bool)
                  }
                  frame True {
                  }
                }
              }
            }
            n101 = Bundle By Name(cluster=w238, "Fire Continues Allowed"=w233) -> (w239:T12)
            n102 = call <vilib>:"Add State(s) to Queue__jki_lib_state_machine.vi"("State(s) in Front (\"\")"=w232, "State(s) in (\"\")"=w236) -> ("States Out"=w235:string)  [unwired: 13 in]
          }
          event "Step size": Value Change {
            n103 = event-data() -> ("NewVal"=w261:dbl)  [unwired: 1 in, 5 out]
            n104 = property on="uangle::1" class="DigNum (strict)"("Increment"=w261) -> ()  [unwired: 2 in, 2 out]
            n105 = property on="vangle::1" class="DigNum (strict)"("Increment"=w261) -> ()  [unwired: 2 in, 2 out]
            n106 = property on="xpos::1" class="DigNum (strict)"("Increment"=w261) -> ()  [unwired: 2 in, 2 out]
            n107 = property on="zpos::1" class="DigNum (strict)"("Increment"=w261) -> ()  [unwired: 2 in, 2 out]
            n108 = property on="wangle::1" class="DigNum (strict)"("Increment"=w261) -> ()  [unwired: 2 in, 2 out]
            n109 = property on="ypos::1" class="DigNum (strict)"("Increment"=w261) -> ()  [unwired: 2 in, 2 out]
          }
          event "Step size 2": Value Change {
            n110 = event-data() -> ("NewVal"=w262:dbl)  [unwired: 1 in, 5 out]
            n111 = control-ref of="Position.Axis 1::33"() -> (w271:refnum<vi>)
            n112 = control-ref of="Position.Axis 1::34"() -> (w267:refnum<vi>)
            n113 = control-ref of="Position.Axis 2::34"() -> (w266:refnum<vi>)
            n114 = control-ref of="Position.Axis 2::33"() -> (w270:refnum<vi>)
            n115 = control-ref of="Position.Axis 4::33"() -> (w268:refnum<vi>)
            n116 = control-ref of="Position.Axis 3::33"() -> (w269:refnum<vi>)
            n117 = control-ref of="Position.Axis 4::34"() -> (w264:refnum<vi>)
            n118 = control-ref of="Position.Axis 3::34"() -> (w265:refnum<vi>)
            n119 = Build Array(w271, w270, w269, w268, w267, w266, w265, w264) -> (w263:refnum<vi>[])
            n120 = for {
              tunnel: w263 -> [w276] mode=indexing
              tunnel: w262 -> [w275]
              n121 = property on="Property Node" class="DigNum (strict)"(reference=w276, "Increment"=w275) -> ()  [unwired: 1 in, 2 out]
            }
          }
          event Value Change {
            n122 = event-data() -> ()  [unwired: 1 in, 6 out]
            n123 = property on="value0::22" class="Bool (strict)"("Val(Sgnl)"=FALSE) -> ()  [unwired: 2 in, 2 out]
          }
          event Panel Close? {
            # "Discard the event because we'll close the front panel ourselves in Macro: Exit"
            # "Close Panel button (pressed) Event\n(this executes Macro: Exit to terminate the VI)"
            n124 = event-data() -> ()  [unwired: 1 in, 1 out]
            n125 = event-data("Discard?"=TRUE) -> ()  [unwired: 1 in, 1 out]
            n126 = call <vilib>:"Add State(s) to Queue__jki_lib_state_machine.vi"("State(s) in Front (\"\")"="Macro: Exit", "State(s) in (\"\")"=w286) -> ("States Out"=w285:string)  [unwired: 13 in]
          }
        }
      }
      frame "---------- Core ----------" {
        # "Do not put any code in this frame.\n(it is a separator no-op)"
        n127 = call <vilib>:"Add State(s) to Queue__jki_lib_state_machine.vi"("State(s) in (\"\")"=w290) -> ("States Out"=w289:string)  [unwired: 14 in]
      }
      frame Default {
        w300 = 42 items=["No error", "Argument error", "Memory is full", "Out of zone", "End of file", "File already open", "Generic file I/O error", "File not found", "File permission error", "Disk is full", "Duplicate path", "Too many files open", "System feature not enabled", "Resource file not found", "Cannot add resource", "Resource not found", "Image not found", "Image memory error", "Pen does not exist", "Config type invalid", "Config token not found", "Config parse error", "Config memory error", "Bad external code format", "Bad external code offset", "External code not present", "Null window", "Destroy window error", "Null menu", "Print aborted", "Bad print record", "Print driver error", "Windows error during printing", "Memory error during printing", "Print dialog error", "Generic print error", "Invalid device refnum", "Device not found", "Device parameter error", "Device unit error", "Cannot open device", "Device call aborted", "Generic error", "Cancelled by user", "Object ID too low", "Object ID too high", "Object not in heap", "Unknown heap", "Unknown object (invalid DefProc)", "Unknown object (DefProc not in table)", "Message out of range", "Invalid (null) method", "Unknown message", "Manager call not supported", "Bad address", "Network operation in progress", "Network operation timed out", "Connection is busy", "Network attribute not supported", "Network error", "Address in use", "System out of memory", "Connection aborted", "Connection refused", "Not connected", "Already connected", "Connection closed", "Initialization error (interapplication manager)", "Bad occurrence", "Wait on unbound occurrence handler", "Occurrence queue overflow", "Datalog type conflict", "Unused", "Unrecognized type (interapplication manager)", "Memory corrupt", "Failed to make temporary DLL", "Old CIN version", "Drag socket not found", "Failed to load drop-object", "Failed to register OLE object", "Failed to release OLE object", "Format specifier type mismatch", "Unknown format specifier", "Too few format specifiers", "Too many format specifiers", "Scan failed", "Newer CIN version", "Error converting to variant", "Runtime menu error", "Password tampered", "Variant attribute not found", "Incompatible variant data type", "Event data is not available", "Event Store is not present", "Occurrence is not found", "Event Queue is not created", "Event info is not available", "Refnum passed is NULL", "Error retrieving Class GUID", "Error retrieving CoClass GUID", "Error retrieving TypeLib GUID.", "Bad built application magic bytes.", "Specific driver is different from the specific driver associated with the Logical Name.", "There is no session opened to the class driver.", "Max Error", "MAX - Error with config objects", "MAX - Error loading configuration", "MAX - Group not supported"]
        # "Current State"
        # "Do not delete, rename, or modify this frame.\n(this is used to capture unhandled states and typos)"
        # "Handle mistyped state name (developer tool)"
        n128 = Format Into String(format string="Software Exception: Unhandled State \"%s\"." ("message"), error in=w296, w291) -> (resulting string=w299:string, error out=w298:errorcluster)  [unwired: 1 in]
        n129 = call <vilib>:"Error Cluster From Error Code.vi"("show call chain? (False)"=TRUE, "error in (no error)"=w298, "error message (\"\")"=w299, "error code (0)"=w300) -> ("error out"=w297:errorcluster)  [unwired: 5 in]
        n130 = call <vilib>:"Add State(s) to Queue__jki_lib_state_machine.vi"("State(s) in (\"\")"=w295) -> ("States Out"=w294:string)  [unwired: 14 in]
      }
      frame "Initialize Core Data" {
        # "Do not delete, rename, or modify this frame.\n(this is used to determine panel behavior on exit)"
        # "originally closed?"
        # "exe?"
        # "If panel starts closed or is an EXE, then close it when we exit"
        n131 = property class="VI"() -> ("Front Panel.Open"=w309:bool)  [unwired: 2 in, 2 out]
        n132 = property class="App"() -> ("App.Kind"=w308:T8)  [unwired: 2 in, 2 out]
        n133 = control-ref of="Current VI Reference"() -> (w302:refnum<vi>)
        n134 = Not(x=w309) -> (.not. x?=w306:bool)
        n135 = Equal?(x=w308, y=T8."Run Time System" ("Application:Kind")) -> (x = y?=w305:bool)
        n136 = Or(x=w306, y=w305) -> (x .or. y?=w303:bool)
        n137 = Bundle By Name(cluster=w304, "Core.Current VI Reference"=w302, "Core.Close Panel on Exit?"=w303) -> (w311:T12)
        n138 = call <vilib>:"Add State(s) to Queue__jki_lib_state_machine.vi"("State(s) in (\"\")"=w313) -> ("States Out"=w312:string)  [unwired: 14 in]
      }
      frame "Error Handler" {
        # "Unhandled Error -- Display it"
        # "Handle any errors here.\nYou can also output any states to clean-up after errors occur"
        # "Clear error"
        n139 = call <vilib>:"General Error Handler.vi"("error in (no error)"=w315) -> ()  [unwired: 10 in, 5 out]
        n140 = call <vilib>:"Add State(s) to Queue__jki_lib_state_machine.vi"("State(s) in Front (\"\")"="/* Post Error States", "State(s) in (\"\")"=w319) -> ("States Out"=w318:string)  [unwired: 13 in]
      }
      frame "Exit" {
        # "Do not put any code in this frame.\n(No errors that occur here will be handled.)"
        n141 = call <vilib>:"Add State(s) to Queue__jki_lib_state_machine.vi"("State(s) in (\"\")"=w324) -> ("States Out"=w323:string)  [unwired: 14 in]
      }
      frame "---------- Data ----------" {
        # "Do not put any code in this frame.\n(It is a separator no-op. You can make a copy of this frame to create a new Data frame)"
        n142 = call <vilib>:"Add State(s) to Queue__jki_lib_state_machine.vi"("State(s) in (\"\")"=w328) -> ("States Out"=w327:string)  [unwired: 14 in]
      }
      frame "Data: Initialize" {
        w329 = FALSE  # Fire Continues Allowed
        w331 = u32 0  # Tik1
        w330 = u32 0  # Tik2
        w332 = FALSE  # Jet trigger
        w333 = 0.0  # Discharge timing offset
        w334 = 0.0  # Heater timing offset
        w335 = T13 {"Current VI Reference"=refnum, "Close Panel on Exit?"=FALSE}  # Core
        # "do not delete - used by framework"
        # "Expand Bundle to add new data elements to shift register data."
        # "Add new data here."
        # "Data names and types of shift register data are defined by this bundle."
        # "Initialize the shift-register data, here.\n(data names are defined by what you wire into the bundle function)"
        n143 = Bundle("Core"=w335, "Heater timing offset"=w334, "Discharge timing offset"=w333, "Jet trigger"=w332, "Tik1"=w331, "Tik2"=w330, "Fire Continues Allowed"=w329) -> (w337:T12)  [unwired: 1 in]
        n144 = call <vilib>:"Add State(s) to Queue__jki_lib_state_machine.vi"("State(s) in (\"\")"=w339) -> ("States Out"=w338:string)  [unwired: 14 in]
      }
      frame "Data: Cleanup" {
        # "Cleanup any data and references, here.\n(this is called automatically, by the Macro: Exit)"
        n145 = Unbundle By Name(w340) -> ("Core.Current VI Reference"=w343:refnum<vi>)
        n146 = Close Reference(reference=w343, error in (no error)=w342) -> (error out=w341:errorcluster)
        n147 = call <vilib>:"Add State(s) to Queue__jki_lib_state_machine.vi"("State(s) in (\"\")"=w345) -> ("States Out"=w344:string)  [unwired: 14 in]
      }
      frame "---------- UI ----------" {
        # "Do not put any code in this frame.\n(It is a separator no-op. You can make a copy of this frame to create a new UI frame)"
        n148 = call <vilib>:"Add State(s) to Queue__jki_lib_state_machine.vi"("State(s) in (\"\")"=w349) -> ("States Out"=w348:string)  [unwired: 14 in]
      }
      frame "UI: Initialize" {
        # "Initialize the User Interface, here.\n(this is called automatically, by the Macro: Init)"
        n149 = call <vilib>:"Add State(s) to Queue__jki_lib_state_machine.vi"("State(s) in (\"\")"=w353) -> ("States Out"=w352:string)  [unwired: 14 in]
      }
      frame "UI: Cursor Set" {
        # "Argument"
        # "Set and Unset Cursor Busy.\n(Usage: \"UI: Cursor Set >> Busy|Idle\")"
        n150 = case shown="\"Idle\", Default" w354 {
          tunnel: w356 -> [w361 w363]
          tunnel: [w360 w362] -> w355
          frame "Idle", Default {
            n151 = call <vilib>:"Unset Busy.vi"("error in (no error)"=w361) -> ("error out"=w360:errorcluster)  [unwired: 10 in]
          }
          frame "Busy" {
            n152 = call <vilib>:"Set Busy.vi"("error in (no error)"=w363) -> ("error out"=w362:errorcluster)  [unwired: 9 in, 1 out]
          }
        }
        n153 = call <vilib>:"Add State(s) to Queue__jki_lib_state_machine.vi"("State(s) in (\"\")"=w359) -> ("States Out"=w358:string)  [unwired: 14 in]
      }
      frame "UI: Front Panel State" {
        # "Argument"
        # "Set Front Panel Open or Closed\n(Usage: \"UI: Front Panel State >> Open|Close\")"
        n154 = Unbundle By Name(w366) -> ("Core.Current VI Reference"=w365:refnum<vi>)
        n155 = case shown="\"Close\"" w364 {
          tunnel: w368 -> [w374 w387]
          tunnel: [w376 w388] -> w367
          tunnel: w365 -> [w375 w385]
          frame "Open", Default {
            n156 = property class="VI"(reference=w375, error in=w374) -> (reference out=w372:refnum<vi>, error out=w373:errorcluster, "Front Panel.Open"=w371:bool)
            n157 = case shown="False" w371 {
              tunnel: [w379 w382] -> w376
              tunnel: w373 -> [w378 w382]
              tunnel: w372 -> [w377 _]
              frame False {
                n158 = invoke class="VI" method="FP.Open"(reference=w377, error in=w378, "Activate"=TRUE, "State"=T9."Standard") -> (error out=w379:errorcluster)  [unwired: 1 in, 4 out]
              }
              frame True {
              }
            }
          }
          frame "Close" {
            n159 = property class="VI"(reference=w385, error in=w387) -> (reference out=w384:refnum<vi>, error out=w386:errorcluster, "Front Panel.Open"=w383:bool)
            n160 = case shown="True" w383 {
              tunnel: [w389 w392] -> w388
              tunnel: w386 -> [w389 w391]
              tunnel: w384 -> [_ w390]
              frame False {
              }
              frame True {
                n161 = invoke class="VI" method="FP.Close"(reference=w390, error in=w391) -> (error out=w392:errorcluster)  [unwired: 1 in, 2 out]
              }
            }
          }
        }
        n162 = call <vilib>:"Add State(s) to Queue__jki_lib_state_machine.vi"("State(s) in (\"\")"=w370) -> ("States Out"=w369:string)  [unwired: 14 in]
      }
      frame "---------- Macro ----------" {
        # "Do not put any code in this frame.\n(It is a separator no-op. You can make a copy of this frame to create a new Macro frame)"
        n163 = call <vilib>:"Add State(s) to Queue__jki_lib_state_machine.vi"("State(s) in (\"\")"=w396) -> ("States Out"=w395:string)  [unwired: 14 in]
      }
      frame "Macro: Initialize" {
        w397 = "Data: Initialize\nInitialize Core Data\nUI: Initialize\nUI: Front Panel State >> Open\nCheck if Fire continues allowed\nInitilize Fire Continues"  # Data: Initialize Initialize Core Data UI: Initialize UI: Front Panel State >> Open Check if Fire continues allowed Initilize Fire Continues
        # "Initialization Macro\n(This is called once, when the VI starts)"
        n164 = call <vilib>:"Add State(s) to Queue__jki_lib_state_machine.vi"("State(s) in Front (\"\")"=w397, "State(s) in (\"\")"=w401) -> ("States Out"=w400:string)  [unwired: 13 in]
      }
      frame "Macro: Exit" {
        # "Exit Macro\n(This is called once, when the VI exits)"
        n165 = Unbundle By Name(w411) -> ("Core.Close Panel on Exit?"=w410:bool)
        n166 = Release Queue(queue=w403, force destroy? (F)=TRUE) -> (error out=w402:errorcluster)  [unwired: 1 in, 2 out]
        n167 = call <vilib>:"Clear Errors.vi"("error in (no error)"=w402) -> ()  [unwired: 5 in, 2 out]
        n168 = Select(t="UI: Front Panel State >> Close", s=w410, f="") -> (s? t:f=w407:string)
        n169 = call <vilib>:"Add State(s) to Queue__jki_lib_state_machine.vi"("State(s) in (\"\")"=w407, "State(s) at Back (\"\")"="Data: Cleanup\nExit") -> ("States Out"=w405:string)  [unwired: 13 in]
        n170 = call <vilib>:"Add State(s) to Queue__jki_lib_state_machine.vi"("State(s) in Front (\"\")"=w405, "State(s) in (\"\")"=w414) -> ("States Out"=w413:string)  [unwired: 13 in]
      }
      frame "---------- New Category ----------" {
        # "Template Separator\n(You can make a copy of, or modify, this frame)"
        n171 = call <vilib>:"Add State(s) to Queue__jki_lib_state_machine.vi"("State(s) in (\"\")"=w418) -> ("States Out"=w417:string)  [unwired: 14 in]
      }
      frame "CheckTimeFire" {
        # "Your code here.\n(You can make a copy of, or modify, this frame)"
        n172 = Unbundle By Name(w425) -> ("Tik1"=w430:u32)
        n173 = Tick Count (ms)() -> (millisecond timer value=w432:u32)
        n174 = Unbundle By Name(w425) -> ("Fire Continues Allowed"=w422:bool)
        n175 = Reciprocal(x="Rate (Hz)") -> (1/x=w421:dbl)
        n176 = Subtract(x=w432, y=w430) -> (x-y=w433:u32)
        n177 = Multiply(x=1000.0, y=w421) -> (x*y=w420:dbl)
        n178 = Greater?(x=w433, y=w420) -> (0:w428:bool)
        n179 = And(x=w428, y="value0::22") -> (x .and. y?=w424:bool)
        n180 = And(x=w422, y=w424) -> (x .and. y?=w423:bool)
        n181 = case shown="True" w423 {
          tunnel: w432 -> [_ w440]
          tunnel: [w438 w440] -> w431
          tunnel: w430 -> [w438 _]
          tunnel: [_ "Action: Fire" ("State(s) in Front (\"\")")] -> w427
          frame False {
          }
          frame True {
          }
        }
        n182 = Bundle By Name(cluster=w425, "Tik1"=w431) -> (w434:T12)
        n183 = call <vilib>:"Add State(s) to Queue__jki_lib_state_machine.vi"("State(s) in Front (\"\")"=w427, "State(s) in (\"\")"=w437) -> ("States Out"=w436:string)  [unwired: 13 in]
        "Fire continues Indicator" <- "value0::22"
      }
      frame "Initilize Fire Continues" {
        # "Your code here.\n(You can make a copy of, or modify, this frame)"
        n184 = Unbundle By Name(w444) -> ("Fire Continues Allowed"=w443:bool)
        n185 = property on="value0::22" class="Bool (strict)"(error in=w446, "Visible"=w443) -> (error out=w445:errorcluster)  [unwired: 1 in, 1 out]
        n186 = Not(x=w443) -> (.not. x?=w441:bool)
        n187 = property on="Fire continues Indicator" class="Bool (strict)"(error in=w445, "Visible"=w441) -> (error out=w442:errorcluster)  [unwired: 1 in, 1 out]
        n188 = call <vilib>:"Add State(s) to Queue__jki_lib_state_machine.vi"("State(s) in (\"\")"=w448) -> ("States Out"=w447:string)  [unwired: 14 in]
      }
      frame "Check if Fire continues allowed" {
        # "Check if it is allowed computer"
        # "Your code here.\n(You can make a copy of, or modify, this frame)"
        n189 = String To IP() -> (0:w456:u32)  [unwired: 1 in]
        n190 = IP To String(1:TRUE ("dot notation? (F)"), 2:w456) -> (0:w457:string)
        n191 = Equal?(x=w457, y="192.168.14.2") -> (x = y?=w451:bool)
        n192 = Not(x=w451) -> (.not. x?=w452:bool)
        n193 = Bundle By Name(cluster=w454, "Fire Continues Allowed"=w451) -> (w453:T12)
        n194 = property on="Allow Fire Continues" class="Bool (strict)"(error in=w450, "Visible"=w452) -> (error out=w449:errorcluster)  [unwired: 1 in, 1 out]
        n195 = call <vilib>:"Add State(s) to Queue__jki_lib_state_machine.vi"("State(s) in (\"\")"=w460) -> ("States Out"=w459:string)  [unwired: 14 in]
      }
      frame "CheckTime2" {
        # "Your code here.\n(You can make a copy of, or modify, this frame)"
        n196 = Unbundle By Name(w469) -> ("Tik2"=w462:u32)
        n197 = Tick Count (ms)() -> (millisecond timer value=w464:u32)
        n198 = Subtract(x=w464, y=w462) -> (x-y=w467:u32)
        n199 = Greater?(x=w467, y=2000) -> (0:w465:bool)
        n200 = case shown="True" w465 {
          tunnel: w464 -> [_ w475]
          tunnel: [w473 w475] -> w463
          tunnel: w462 -> [w473 _]
          tunnel: [_ "Action: update expt vars"] -> w461
          frame False {
          }
          frame True {
          }
        }
        n201 = Bundle By Name(cluster=w469, "Tik2"=w463) -> (w468:T12)
        n202 = call <vilib>:"Add State(s) to Queue__jki_lib_state_machine.vi"("State(s) in Front (\"\")"=w461, "State(s) in (\"\")"=w472) -> ("States Out"=w471:string)  [unwired: 13 in]
      }
      frame "Action: Fire" {
        n203 = property on="fire::10" class="Str"(error in=w477, "Val(Sgnl)"="fire>>force" ("Value (Signaling)")) -> (error out=w476:errorcluster)  [unwired: 1 in, 1 out]
        n204 = call <vilib>:"Add State(s) to Queue__jki_lib_state_machine.vi"("State(s) in (\"\")"=w481) -> ("States Out"=w480:string)  [unwired: 14 in]
      }
      frame "Action: MoveCap" {
        n205 = local read "ypos::1"() -> (w496:dbl)
        n206 = case shown="\"In\"" w492 {
          tunnel: [25.0 ("Value (Signaling)") 0.0 ("Value (Signaling)")] -> w491
          tunnel: [-20.0 ("x") 20.0 ("x")] -> w490
          frame "In" {
          }
          frame "Out", Default {
          }
        }
        n207 = Add(x=w490, y=w496) -> (x+y=w495:dbl)
        n208 = property on="ypos::1" class="DigNum (strict)"(error in=w494, "Val(Sgnl)"=w495) -> (error out=w493:errorcluster)  [unwired: 1 in, 1 out]
        n209 = property on="EnableMotor::6" class="Bool (strict)"("Val(Sgnl)"=TRUE ("Value (Signaling)")) -> (error out=w488:errorcluster)  [unwired: 2 in, 1 out]
        n210 = call <userlib>:"Wait (ms)__ogtk.vi"("error in (no error)"=w488, "milliseconds to wait"=u32 1000) -> ("error out"=w487:errorcluster)  [unwired: 8 in, 1 out]
        n211 = property on="position::4" class="DigNum (strict)"(error in=w487, "Val(Sgnl)"=w491) -> (error out=w484:errorcluster)  [unwired: 1 in, 1 out]
        n212 = call <userlib>:"Wait (ms)__ogtk.vi"("error in (no error)"=w484, "milliseconds to wait"=u32 6000) -> ("error out"=w482:errorcluster)  [unwired: 8 in, 1 out]
        n213 = property on="EnableMotor::6" class="Bool (strict)"(error in=w482, "Val(Sgnl)"=FALSE ("Value (Signaling)")) -> ()  [unwired: 1 in, 2 out]
        n214 = call <vilib>:"Add State(s) to Queue__jki_lib_state_machine.vi"("State(s) in (\"\")"=w499) -> ("States Out"=w498:string)  [unwired: 14 in]
      }
      frame "Action: update expt vars" {
        # "Your code here.\n(You can make a copy of, or modify, this frame)"
        n215 = call "SQL Server Info.vi"() -> ("SQL Server Info"=w516:T15)
        n216 = call "SQL Query.vi"("SQL Server Info"=w516, "Query"="SELECT id, expt_device_id, variablename, `get`, `set`, `defaultvalue`, `startvalue`, `endvalue` FROM expt_device_variable WHERE  variablename in('ipaddress','position','bigshutterposition','smallshutterposition','bigshuttermode','smallshuttermode'\r\n)AND expt_device_id = '179' GROUP BY id;" ("Device ID")) -> ("data"=w506:string[][])  [unwired: 8 in, 1 out]
        n217 = Index Array(array=w506, index (col)=2 ("disabled index (col)")) -> (element=w505:string[])  [unwired: 1 in]
        n218 = Search 1D Array(1D array=w505, element="smallshuttermode") -> (index of element=w509:i32)  [unwired: 1 in]
        n219 = Search 1D Array(1D array=w505, element="bigshuttermode") -> (index of element=w510:i32)  [unwired: 1 in]
        n220 = Index Array(array=w506, index (row)=w509, index (col)=6 ("disabled index (col)")) -> (element=→"PWshutter Scanstart":string)
        n221 = Index Array(array=w506, index (row)=w510, index (col)=6 ("disabled index (col)")) -> (element=→"Heater Scanstart":string)
        n222 = call <vilib>:"Add State(s) to Queue__jki_lib_state_machine.vi"("State(s) in (\"\")"=w520) -> ("States Out"=w519:string)  [unwired: 14 in]
      }
    }
  }
  n223 = disable-structure shown="Disabled" {
    frame Disabled {
      n224 = call "DefaultValue_Variable_MC.vi"() -> ()  [unwired: 4 in]
    }
    frame Enabled {
    }
  }
  n225 = disable-structure shown="Disabled" {
    frame Disabled {
      n226 = call "SQL edit expt device variable.vi"("Variable Name"="bigshuttermode", "Device ID"="179", "Corresponding values"=string[] ["Manual"], "Columns"=string[] ["startvalue"]) -> ()  [unwired: 7 in, 1 out]
    }
    frame Enabled {
    }
  }
  n227 = disable-structure shown="Disabled" {
    frame Disabled {
    }
    frame Enabled {
    }
  }
  n228 = disable-structure shown="Disabled" {
    frame Disabled {
      n229 = call <vilib>:"Application Directory.vi"() -> ("Application Directory"=w528:path)
      n230 = call <vilib>:"Application Directory.vi"() -> ("Application Directory"=w532:path)
      n231 = Build Path(base path=w528, name or relative path="Heater_Timing_Offset.txt") -> (appended path=w529:path)
      n232 = Build Path(base path=w532, name or relative path="Discharge_Timing_Offset.txt") -> (appended path=w533:path)
      n233 = Number To Exponential String(number="Offset Heater timing") -> (E-format string=w526:string)  [unwired: 3 in]
      n234 = Number To Exponential String(number="Offset discharge timing") -> (E-format string=w534:string)  [unwired: 3 in]
      n235 = Write to Text File(file (use dialog)=w529, text=w526) -> ()  [unwired: 2 in, 3 out]
      n236 = Write to Text File(file (use dialog)=w533, text=w534) -> ()  [unwired: 2 in, 3 out]
      n237 = call <vilib>:"Application Directory.vi"() -> ("Application Directory"=w542:path)
      n238 = call <vilib>:"Application Directory.vi"() -> ("Application Directory"=w538:path)
      n239 = Build Path(base path=w542, name or relative path="Heater_Timing_Offset.txt") -> (appended path=w543:path)
      n240 = Build Path(base path=w538, name or relative path="Discharge_Timing_Offset.txt") -> (appended path=w537:path)
      n241 = Read from Text File(file (use dialog)=w543) -> (text=w540:string)  [unwired: 3 in, 3 out]
      n242 = Fract/Exp String To Number(string=w540) -> (number=w544:dbl)  [unwired: 3 in, 1 out]
      n243 = Read from Text File(file (use dialog)=w537) -> (text=w539:string)  [unwired: 3 in, 3 out]
      n244 = Fract/Exp String To Number(string=w539) -> (number=w535:dbl)  [unwired: 3 in, 1 out]
      n245 = property on="Offset Heater timing" class="DigNum (strict)"("Val(Sgnl)"=w544) -> ()  [unwired: 2 in, 2 out]
      n246 = property on="Offset discharge timing" class="DigNum (strict)"("Val(Sgnl)"=w535) -> ()  [unwired: 2 in, 2 out]
    }
    frame Enabled {
    }
  }
